vi "Z900_navX_SPI_Read.vi"(8 "error in (no error)":errorcluster, 10 "Registry":u8[](array[numeric]), 11 "Interface TypeDefs":T1 {"I2CDevRef"."Device Address" format="%.0x"}) -> (0 "error out":errorcluster, 1 "Valid":bool, 2 "Registry":u8[](array[numeric]), 3 "Interface TypeDefs":T1 {"I2CDevRef"."Device Address" format="%.0x"})   [LabVIEW 2015, in "navX Library v2.lvlib"]
uses:
  navX Library v2.lvlib
  TypeDefs/Z900_navX_InterfaceTypeDef.ctl
  <vilib>/Rock Robotics/WPI/SerialPort/WPI_SerialPortRef.ctl
  <vilib>/Rock Robotics/WPI/I2C/WPI_I2CDevRef.ctl
  <vilib>/Rock Robotics/SystemInterfaces/i2clib/i2c_bus.ctl
  <vilib>/Rock Robotics/WPI/SPI/WPI_SPIDevRef.ctl
  <vilib>/Rock Robotics/SystemInterfaces/spilib/spi_bus.ctl
  TypeDefs/Z900_navX_DeviceRegisters.ctl
  TypeDefs/Flags/Z900_navX_Flags_CapabilityTypeDef.ctl
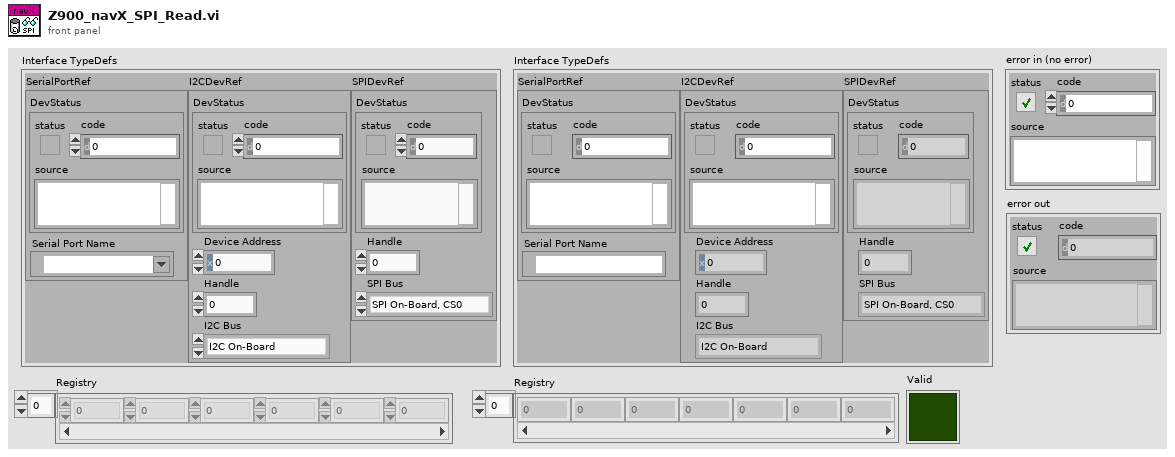
[diagram p1: front panel]
types:
  T1 = typedef "navX Library v2.lvlib/Z900_navX_InterfaceTypeDef.ctl" = cluster{"SerialPortRef":T2, "I2CDevRef":T3, "SPIDevRef":T5}
  T2 = typedef "WPI_SerialPortRef.ctl" = cluster{"DevStatus":errorcluster, "Serial Port Name":refnum<visa-resource-name>}
  T3 = typedef "WPI_I2CDevRef.ctl" = cluster{"DevStatus":errorcluster, "Device Address":u8, "Handle":i32, "I2C Bus":T4}
  T4 = typedef "i2c_bus.ctl" = enum16{"I2C On-Board", "I2C MXP", "Invalid"}
  T5 = typedef "WPI_SPIDevRef.ctl" = cluster{"DevStatus":errorcluster, "Handle":i32, "SPI Bus":T6}
  T6 = typedef "spi_bus.ctl" = enum16{"SPI On-Board, CS0", "SPI On-Board, CS1", "SPI On-Board, CS2", "SPI On-Board, CS3", "SPI MXP", "Invalid"}
  T7 = typedef "navX Library v2.lvlib/Z900_navX_DeviceRegisters.ctl" = u8
  T8 = typedef "navX Library v2.lvlib/Z900_navX_Flags_CapabilityTypeDef.ctl" = u16
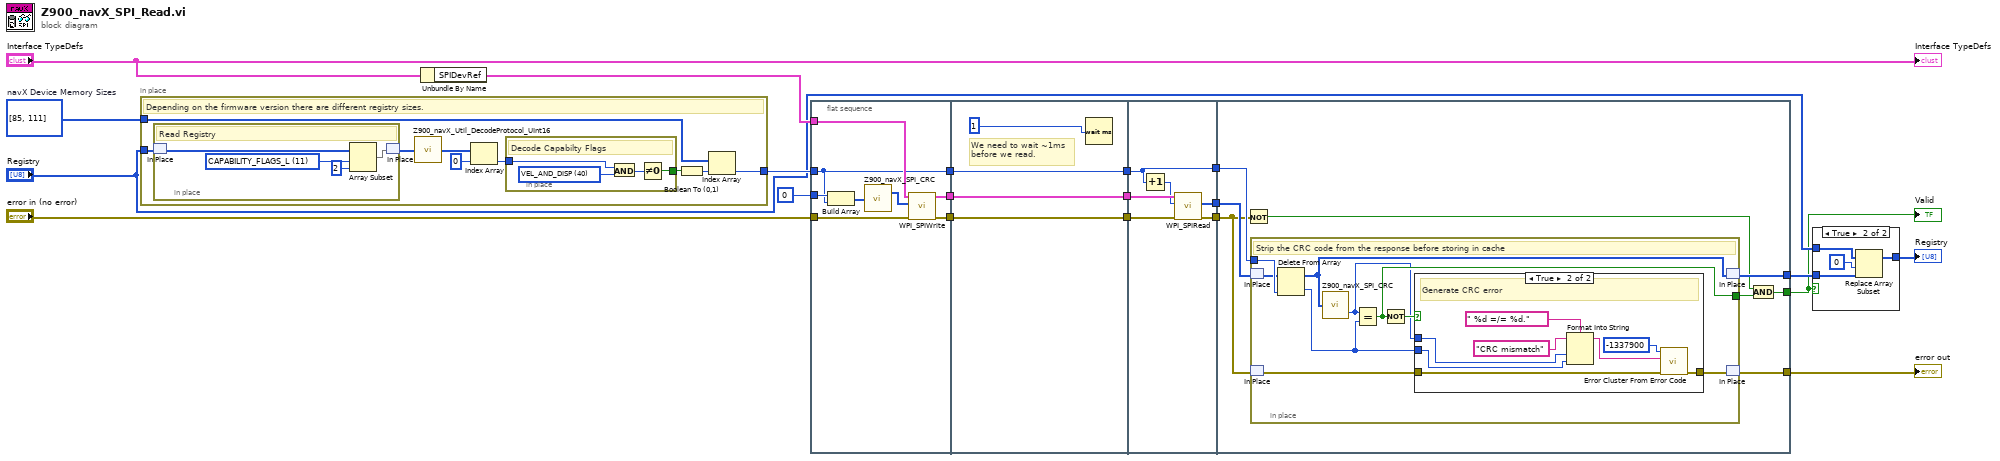
[diagram p0: block diagram]
diagram:
  w7 = i32[] [85, 111]  # navX Device Memory Sizes
  n1 = in-place {
    in-place-border: "Registry" -> [w29]
    in-place-border: w7 -> [w22]
    in-place-border: [w21] -> w8
    # "Depending on the firmware version there are different registry sizes."
    n2 = in-place {
      w37 = T7 11 items=["WHOAMI"=0, "HW_REV"=1, "FW_VER_MAJOR"=2, "FW_VER_MINOR"=3, "UPDATE_RATE_HZ"=4, "ACCEL_FSR_G"=5, "GYRO_FSR_DPS"=6, "OP_STATUS"=8, "CAL_STATUS"=9, "SELFTEST_STATUS"=10, "CAPABILITY_FLAGS_L"=11, "CAPABILITY_FLAGS_H"=12, "SENSOR_STATUS"=16, "TIMESTAMP"=18, "YAW"=22, "ROLL"=24, "PITCH"=26, "HEADING"=28, "FUSED_HEADING"=30, "ALTITUDE_I"=32, "ALTITUDE_D"=34, "LINERA_ACC_X"=36, "LINERA_ACC_Y"=38, "LINERA_ACC_Z"=40, "QUAT_W"=42, "QUAT_X"=44, "QUAT_Y"=46, "QUAT_Z"=48, "MPU_TEMP_C"=50, "GYRO_X"=52, "GYRO_Y"=54, "GYRO_Z"=56, "ACC_X"=58, "ACC_Y"=60, "ACC_Z"=62, "MAG_X"=64, "MAG_Y"=66, "MAG_Z"=68, "PRESSURE_I"=70, "PRESSURE_D"=72, "PRESSURE_TEMP"=74, "YAW_OFFSET"=76, "QUAT_OFFSET_W"=78, "QUAT_OFFSET_X"=80, "QUAT_OFFSET_Y"=82, "QUAT_OFFSET_Z"=84, "INTEGRATION_CONTROL"=86, "VELOCITY_X"=88, "VELOCITY_Y"=92, "VELOCITY_Z"=96, "DISPLACMENT_X"=100, "DISPLACMENT_Y"=104, "DISPLACEMENT_Z"=108] ("Device Register")
      # "Read Registry"
      n3 = in-place-match #1(w29) -> (w35:u8[])
      n4 = Array Subset(array=w35, index=w37, length=2) -> (w36:u8[])
      n5 = in-place-match #1(w36) -> (w26:u8[])
    }
    n6 = call "Z900_navX_Util_DecodeProtocol_UInt16.vi"("Little Endian"=w26) -> ("UInt16"=w27:u16[])
    n7 = Index Array(array=w27, index=0) -> (element=w25:u16)
    n8 = in-place {
      in-place-border: w25 -> [w31]
      in-place-border: [w30] -> w24
      w33 = T8 40 items=["OMNIMOUNT"=4, "OMNIMOUNT_CONFIG_MASK"=38, "VEL_AND_DISP"=40, "YAW_RESET"=80] ("Capability Flag")
      # "Decode Capabilty Flags"
      n9 = And(x=w31, y=w33) -> (x .and. y?=w32:T8)
      n10 = Not Equal To 0?(x=w32) -> (x != 0?=w30:bool)
    }
    n11 = Boolean To (0,1)(Boolean=w24) -> (0, 1=w23:i16)
    n12 = Index Array(array=w22, index=w23) -> (element=w21:i32)
  }
  n13 = Unbundle By Name("Interface TypeDefs") -> ("SPIDevRef"=w9:T5)
  n14 = flat-sequence {
    tunnel: u8 0 ("hex") -> [w45]
    tunnel: w8 -> [w40]
    tunnel: w9 -> [w42]
    tunnel: [w41] -> w20
    tunnel: [w40] -> w19
    tunnel: [w39] -> w18
    tunnel: "error in (no error)" -> [w38]
    tunnel: w20 -> [w48]
    tunnel: [w48] -> w17
    tunnel: [w47] -> w16
    tunnel: w19 -> [w47]
    tunnel: w18 -> [w46]
    tunnel: [w46] -> w15
    tunnel: w17 -> [w55]
    tunnel: w16 -> [w52]
    tunnel: [w53] -> w14
    tunnel: [w52] -> w13
    tunnel: w15 -> [w51]
    tunnel: [w50] -> w12
    tunnel: w14 -> [w60]
    tunnel: w13 -> [w63]
    tunnel: [w61] -> w4
    tunnel: [w59] -> w11
    tunnel: w12 -> [w57]
    tunnel: [w56] -> w1
    frame #0 {
      n15 = Build Array(w45, w40) -> (w44:i32[])
      n16 = call "Z900_navX_SPI_CRC.vi"("Message"=w44) -> ("Message with CRC"=w43:u8[])  [unwired: 1 out]
      n17 = call <vilib>:"WPI_SPIWrite.vi"("error in (no error)"=w38, "Data To Send"=w43, "SPIDevRef"=w42) -> ("error out"=w39:errorcluster, "SPIDevRef"=w41:T5)  [unwired: 6 in, 1 out]
    }
    frame #1 {
      # "We need to wait ~1ms\nbefore we read."
      n18 = Wait (ms)(milliseconds to wait=u32 1) -> ()  [unwired: 1 out]
    }
    frame #2 {
      n19 = Increment(x=w52) -> (x+1=w54:i32)
      n20 = call <vilib>:"WPI_SPIRead.vi"("error in (no error)"=w51, "Num to Read"=w54, "SPIDevRef"=w55) -> ("error out"=w50:errorcluster, "Received Data"=w53:u8[])  [unwired: 6 in, 1 out]
    }
    frame #3 {
      n21 = Not(x=w57) -> (.not. x?=w58:bool)
      n22 = in-place {
        in-place-border: w63 -> [w72]
        in-place-border: [w69] -> w62
        # "Strip the CRC code from the response before storing in cache"
        n23 = in-place-match #2(w60) -> (w71:u8[])
        n24 = in-place-match #3(w57) -> (w64:errorcluster)
        n25 = Delete From Array(array=w71, index=w72) -> (deleted portion=w66:u8, array with subset deleted=w70:u8[])  [unwired: 1 in]
        n26 = call "Z900_navX_SPI_CRC.vi"("Message"=w70) -> ("CRC"=w67:u8)  [unwired: 1 out]
        n27 = Equal?(x=w67, y=w66) -> (x = y?=w69:bool)
        n28 = Not(x=w69) -> (.not. x?=w68:bool)
        n29 = case shown="True" w68 {
          tunnel: w67 -> [_ w79]
          tunnel: w66 -> [_ w78]
          tunnel: w64 -> [w73 w75]
          tunnel: [w73 w74] -> w65
          frame False {
          }
          frame True {
            # "Generate CRC error"
            n30 = Format Into String(format string=" %d =/= %d.", initial string="CRC mismatch", w79, w78) -> (resulting string=w76:string)  [unwired: 1 in, 1 out]
            n31 = call <vilib>:"Error Cluster From Error Code.vi"("error in (no error)"=w75, "error message (\"\")"=w76, "error code (0)"=-1337900 ("code")) -> ("error out"=w74:errorcluster)  [unwired: 6 in]
          }
        }
        n32 = in-place-match #2(w70) -> (w59:u8[])
        n33 = in-place-match #3(w65) -> (w56:errorcluster)
      }
      n34 = And(x=w58, y=w62) -> (x .and. y?=w61:bool)
    }
  }
  n35 = case shown="True" w4 {
    tunnel: "Registry" -> [w82 w86]
    tunnel: [w82 w85] -> w5
    tunnel: w11 -> [_ w84]
    frame False {
    }
    frame True {
      n36 = Replace Array Subset(array=w86, new element=w84, index=u8 0 ("hex")) -> (w85:u8[])
    }
  }
  "Registry" <- w5
  "Interface TypeDefs" <- "Interface TypeDefs"
  "Valid" <- w4
  "error out" <- w1
